vi "Read D-Register.vi"() -> ()   [LabVIEW 2017]
uses:
  <instrlib>/Samwontech TEMP2xxx/Samwontech TEMP2xxx.lvlib
panel:
  out "Data Valid":bool
  in  "D-register number":u32
  out "Data":u32
  in  "VISA resource name":refnum<visa-resource-name>
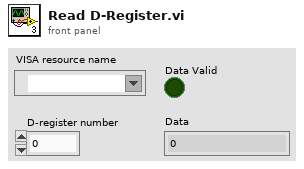
[diagram p1: front panel]
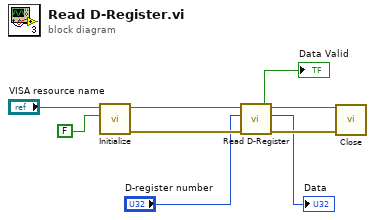
[diagram p0: block diagram]
diagram:
  n1 = call <instrlib>:"Initialize.vi"("ID Query (True)"=FALSE, "VISA resource name"="VISA resource name") -> ("error out"=w6:errorcluster, "VISA resource name out"=w7:refnum<visa-resource-name>)  [unwired: 8 in]
  n2 = call <instrlib>:"Read D-Register.vi"("error in"=w6, "D-register number"="D-register number", "VISA resource name"=w7) -> ("error out"=w4:errorcluster, "Data"=→"Data":u32, "VISA resource name out"=w5:refnum<visa-resource-name>, "Data Valid"=→"Data Valid":bool)  [unwired: 5 in]
  n3 = call <instrlib>:"Close.vi"("error in (no error)"=w4, "VISA resource name"=w5) -> ()  [unwired: 9 in, 1 out]
